vi "Teleop.vi"(10 "Match Info":T1={"Autonomous Elapsed Seconds"=0.0, "TeleOp Elapsed Seconds"=0.0, "Disabled Elapsed Seconds"=0.0, "Visited Autonomous"=FALSE, "Visited TeleOp"=FALSE, "Visited Disabled"=FALSE, "Autonomous Settings"={"Autonomous Style"=enum."Independent", "VI Refnum"=refnum}}, 11 "Call Context":T2) -> ()   [LabVIEW 2018]
doc: "This VI is called for each TeleOp packet received from the DS where the robot is not disabled. It is often used to read from the joysticks and update I/O or to update setpoints for timed control loops. It should complete and return within 20 milliseconds or it may miss DS packets."
uses:
  <vilib>/Rock Robotics/WPI/DriverStation/WPI_DriverStationDerivedRobotMode.ctl
  <vilib>/Rock Robotics/WPI/DriverStation/WPI_DriverStationMatch Info.ctl
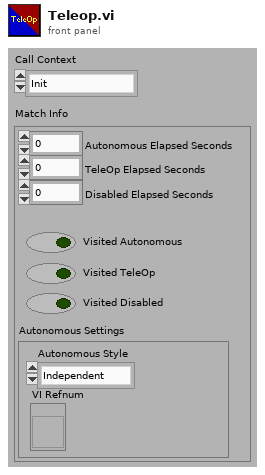
[diagram p1: front panel]
types:
  T1 = typedef "WPI_DriverStationMatch Info.ctl" = cluster{"Autonomous Elapsed Seconds":dbl, "TeleOp Elapsed Seconds":dbl, "Disabled Elapsed Seconds":dbl, "Visited Autonomous":bool, "Visited TeleOp":bool, "Visited Disabled":bool, "Autonomous Settings":cluster{"Autonomous Style":enum16{"Iterative", "Independent"}, "VI Refnum":refnum<vi>}}
  T2 = typedef "WPI_DriverStationDerivedRobotMode.ctl" = enum16{"Init", "Execute", "Stop"}
  T3 = typedef "ADIS Gyro Values.ctl" = cluster{"IMU Data Out":cluster{"X Gyro (°/sec)":dbl, "Y Gyro (°/sec)":dbl, "Z Gyro (°/sec)":dbl, "X Accel (g)":dbl, "Y Accel (g)":dbl, "Z Accel (g)":dbl, "X Mag(mgauss)":dbl, "Y Mag(mgauss)":dbl, "Z Mag(mgauss)":dbl, "Pressure(mbar)":dbl, "Temp(C)":dbl}, "IMU Angle Delta":cluster{"X":dbl, "Y":dbl, "Z":dbl}, "IMU AHRS":cluster{"Pitch":dbl, "Roll":dbl, "Yaw":dbl}}
  T4 = typedef "DriveJoystickButtonMapping.ctl" = cluster{"relative encoders?":bool, "zero relative encoder":bool, "reset field orientation":bool, "use field orientation":bool}
  T5 = typedef "Robot Pivot Motion Commands.ctl" = cluster{"Front Right":T6, "Front Left":T6, "Rear Left":T6, "Rear Right":T6, "Drive Mode":T7}
  T6 = typedef "Pivot Motor Commands.ctl" = cluster{"Drive Power":dbl, "Drive Distance (in)":dbl, "Steer Power":dbl, "Steer Angle (deg)":dbl, "Steer Angle Error (deg)":dbl}
  T7 = typedef "Robot Drive Mode.ctl" = enum16{"Velocity", "Distance"}
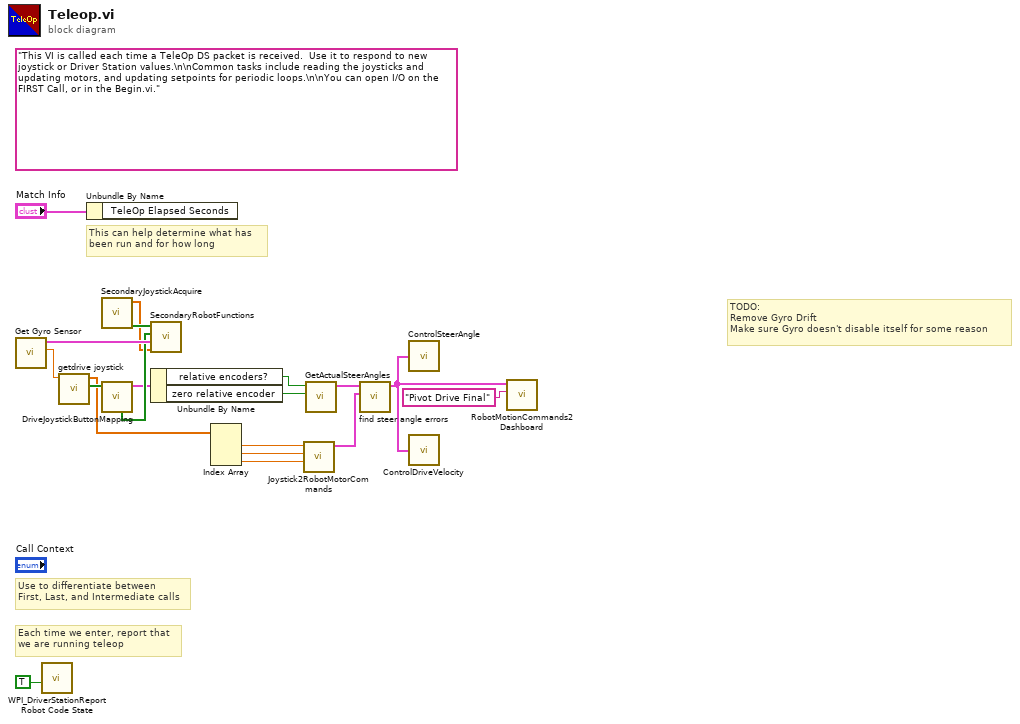
[diagram p0: block diagram]
diagram:
  (unwired) "This VI is called each time a TeleOp DS packet is received.  Use it to respond to new joystick or Driver Station values.\n\nCommon tasks include reading the joysticks and updating motors, and updating setpoints for periodic loops.\n\nYou can open I/O on the FIRST Call, or in the Begin.vi."
  # "TODO:\nRemove Gyro Drift\nMake sure Gyro doesn't disable itself for some reason"
  # "Each time we enter, report that\nwe are running teleop"
  # "Use to differentiate between\nFirst, Last, and Intermediate calls"
  # "This can help determine what has\nbeen run and for how long"
  n1 = call "Get Gyro Sensor.vi"() -> ("Robot Field Orientation (deg)"=w13:dbl, "ADIS Gyro Values"=w16:T3)  [unwired: 10 in]
  n2 = call <vilib>:"WPI_DriverStationReport Robot Code State.vi"("TeleOp"=TRUE ("Autonomous")) -> ()  [unwired: 10 in, 1 out]
  n3 = call "getdrive joystick.vi"("Robot filed orientation (deg)"=w13) -> ("drive joystick buttons"=w12:bool[], "drive joystick values"=w11:dbl[])  [unwired: 9 in]
  n4 = Unbundle By Name("Match Info") -> ()  [unwired: 1 out]
  n5 = call "SecondaryJoystickAcquire.vi"() -> ("Secondary Joystick Buttons"=w17:bool[], "Secondary Joystick Values"=w14:dbl[])  [unwired: 10 in]
  n6 = call "DriveJoystickButtonMapping.vi"("drive joystick buttons"=w12) -> ("DriveJoystickButtonMapping"=w7:T4, "drive joystick buttons indicator"=w15:bool[])  [unwired: 9 in]
  n7 = call "SecondaryRobotFunctions.vi"("Secondary Joystick Values"=w14, "ADIS Gyro Values"=w16, "Drive Joystick Buttons"=w15, "Secondary Joystick Buttons"=w17) -> ()  [unwired: 8 in]
  n8 = Unbundle By Name(w7) -> ("relative encoders?"=w6:bool, "zero relative encoder"=w5:bool)
  n9 = Index Array(array=w11) -> (element #1=w10:dbl, element #2=w9:dbl, element #3=w8:dbl)  [unwired: 3 in]
  n10 = call "Joystick2RobotMotorCommands.vi"("Joystick R"=w8, "Joystick Y"=w9, "Joystick X"=w10) -> ("Robot Motion Commands"=w2:T5)  [unwired: 8 in]
  n11 = call "GetActualSteerAngles.vi"("Zero Relative Encoder"=w5, "Relative Encoders?"=w6) -> ("Robot Motion Commands"=w1:T5)  [unwired: 9 in]
  n12 = call "find steer angle errors.vi"("Desired Motion"=w2, "Actual Angles"=w1) -> ("Commanded Motion"=w4:T5)  [unwired: 9 in]
  n13 = call "ControlSteerAngle.vi"("Robot Motion Commands"=w4) -> ()
  n14 = call "ControlDriveVelocity.vi"("Robot Motion Commands"=w4) -> ()
  n15 = call "RobotMotionCommands2Dashboard.vi"("Label"="Pivot Drive Final", "Robot Motion Commands"=w4) -> ()  [unwired: 10 in]
